vi "VerticalLinearIndicator.vi"(8 "FixedMarkers":dbl[](array[numeric]), 9 "Value":dbl, 10 "SizeAndLocation":T2, 11 "Refnum in":T1) -> (3 "Refnum out":T1)   [LabVIEW 2015]
uses:
  <vilib>/vision/Image Controls.llb/IMAQ Image.ctl
panel:
  in  "Group":string
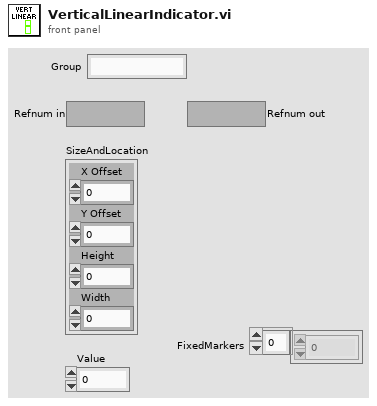
[diagram p1: front panel]
types:
  T1 = typedef "IMAQ Image.ctl" = refnum<image>
  T2 = cluster{"X Offset":i32, "Y Offset":i32, "Height":i32, "Width":i32}
  T3 = cluster{"Left":i32, "Top":i32, "Right":i32, "Bottom":i32}
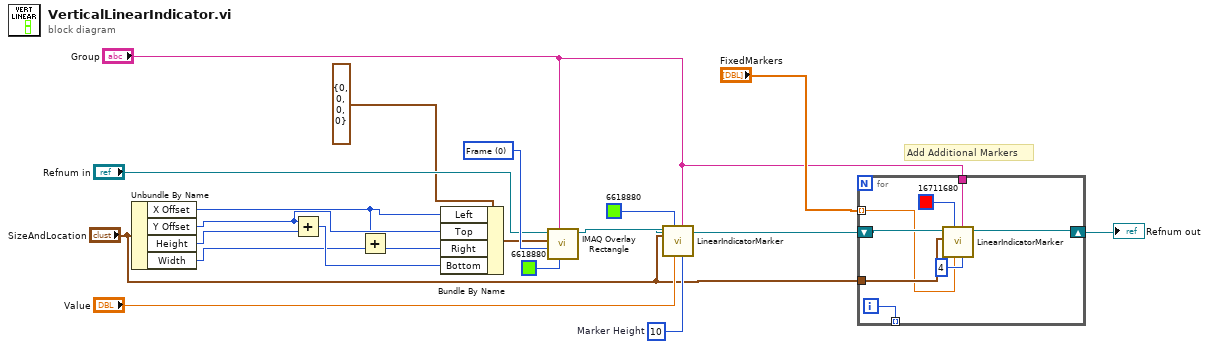
[diagram p0: block diagram]
diagram:
  w19 = 10  # Marker Height
  w15 = u32 0 items=["Frame", "Fill", "Highlight"] ("Drawing Mode (Frame)")
  # "Add Additional Markers"
  n1 = Unbundle By Name("SizeAndLocation") -> ("X Offset"=w7:i32, "Y Offset"=w20:i32, "Height"=w17:i32, "Width"=w9:i32)
  n2 = Add(x=w20, y=w17) -> (x+y=w14:i32)
  n3 = Add(x=w7, y=w9) -> (x+y=w8:i32)
  n4 = Bundle By Name(cluster=T3 {"Left"=0, "Top"=0, "Right"=0, "Bottom"=0} ("Rectangle"), "Left"=w7, "Top"=w20, "Right"=w8, "Bottom"=w14) -> (w13:T3)
  n5 = call "IMAQ Overlay Rectangle"("Color"=u32 6618880, "Group"="Group", "Drawing Mode (Frame)"=w15, "Rectangle"=w13, "Image"="Refnum in") -> ("Image Out"=w6:T1)  [unwired: 5 in, 1 out]
  n6 = call "LinearIndicatorMarker.vi"("Marker Height"=w19, "Group"="Group", "Value"="Value", "Color"=u32 6618880, "RectangleSizeAndLocation"="SizeAndLocation", "Image"=w6) -> ("Image Out"=w5:T1)  [unwired: 5 in]
  n7 = for {
    shift-right: [w27] -> w11
    shift-left: w5 -> [w28]
    tunnel: "SizeAndLocation" -> [w26]
    tunnel: [w23] -> _ mode=indexing
    tunnel: "FixedMarkers" -> [w22] mode=indexing
    tunnel: "Group" -> [w21]
    i -> [w23]
    n8 = call "LinearIndicatorMarker.vi"("Marker Height"=4, "Group"=w21, "Value"=w22, "Color"=u32 16711680, "RectangleSizeAndLocation"=w26, "Image"=w28) -> ("Image Out"=w27:T1)  [unwired: 5 in]
  }
  "Refnum out" <- w11
